vi "RT Video Server.vi"(11 "reader url":string) -> ()   [LabVIEW 2015]
uses:
  Controls/RT Streamer Queue element.ctl
  Controls/RT Streamer State.ctl
  RT Controls/Generic instruction typedef.ctl
  LP Globals.vi
  <vilib>/vision/NI_Vision_Development_Module.lvlib
  <resource>/objmgr/ni.dex.rc
  <vilib>/vision/Image Controls.llb/IMAQ Image.ctl
  IP Dev Area/IP results.ctl
panel:
  in  "Frames":u16
  in  "StartSave":bool
  out "error out":errorcluster
  out "output cluster":T1
  out "Frame Rate":dbl
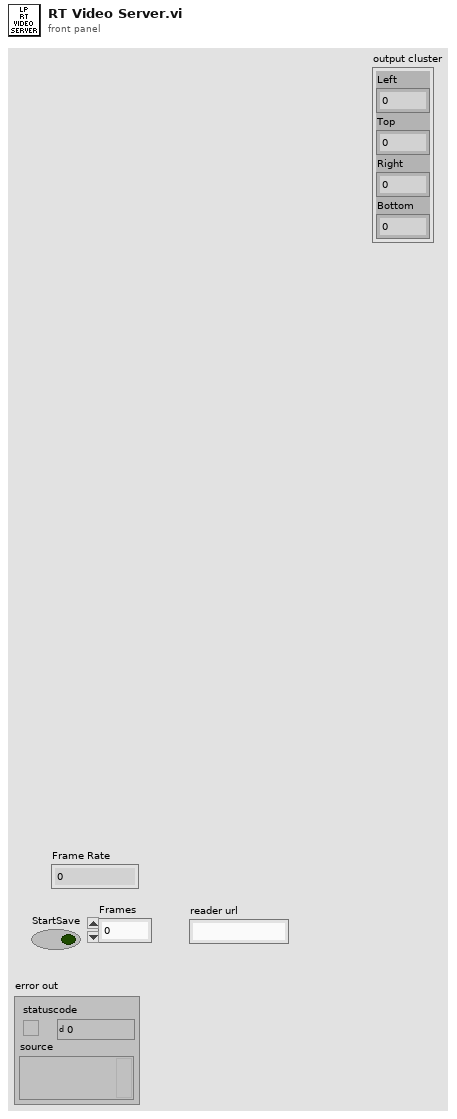
[diagram p1: front panel]
types:
  T1 = cluster{"Left":i32, "Top":i32, "Right":i32, "Bottom":i32}
  T2 = typedef "Image Type" = u32
  T3 = typedef "RT Streamer Queue element.ctl" = cluster{"CMD":T4, "Data":variant, "Error in":errorcluster}
  T4 = typedef "RT Streamer State.ctl" = enum16{"Init", "Idle", "Stream", "Listen", "SetRefrashRate", "SendCmdAck", "SendCmdDone", "SendSysState", "StartRecord", "Green Cordinates", "Error"}
  T5 = typedef "IMAQ Image.ctl" = refnum<image>
  T6 = typedef "Generic instruction typedef.ctl" = cluster{"CMD":string, "Data":variant}
  T7 = typedef "IP results.ctl" = cluster{"X":u16, "Y":u16, "A":dbl, "B":dbl, "Grade":u16, "Frame#":u16}
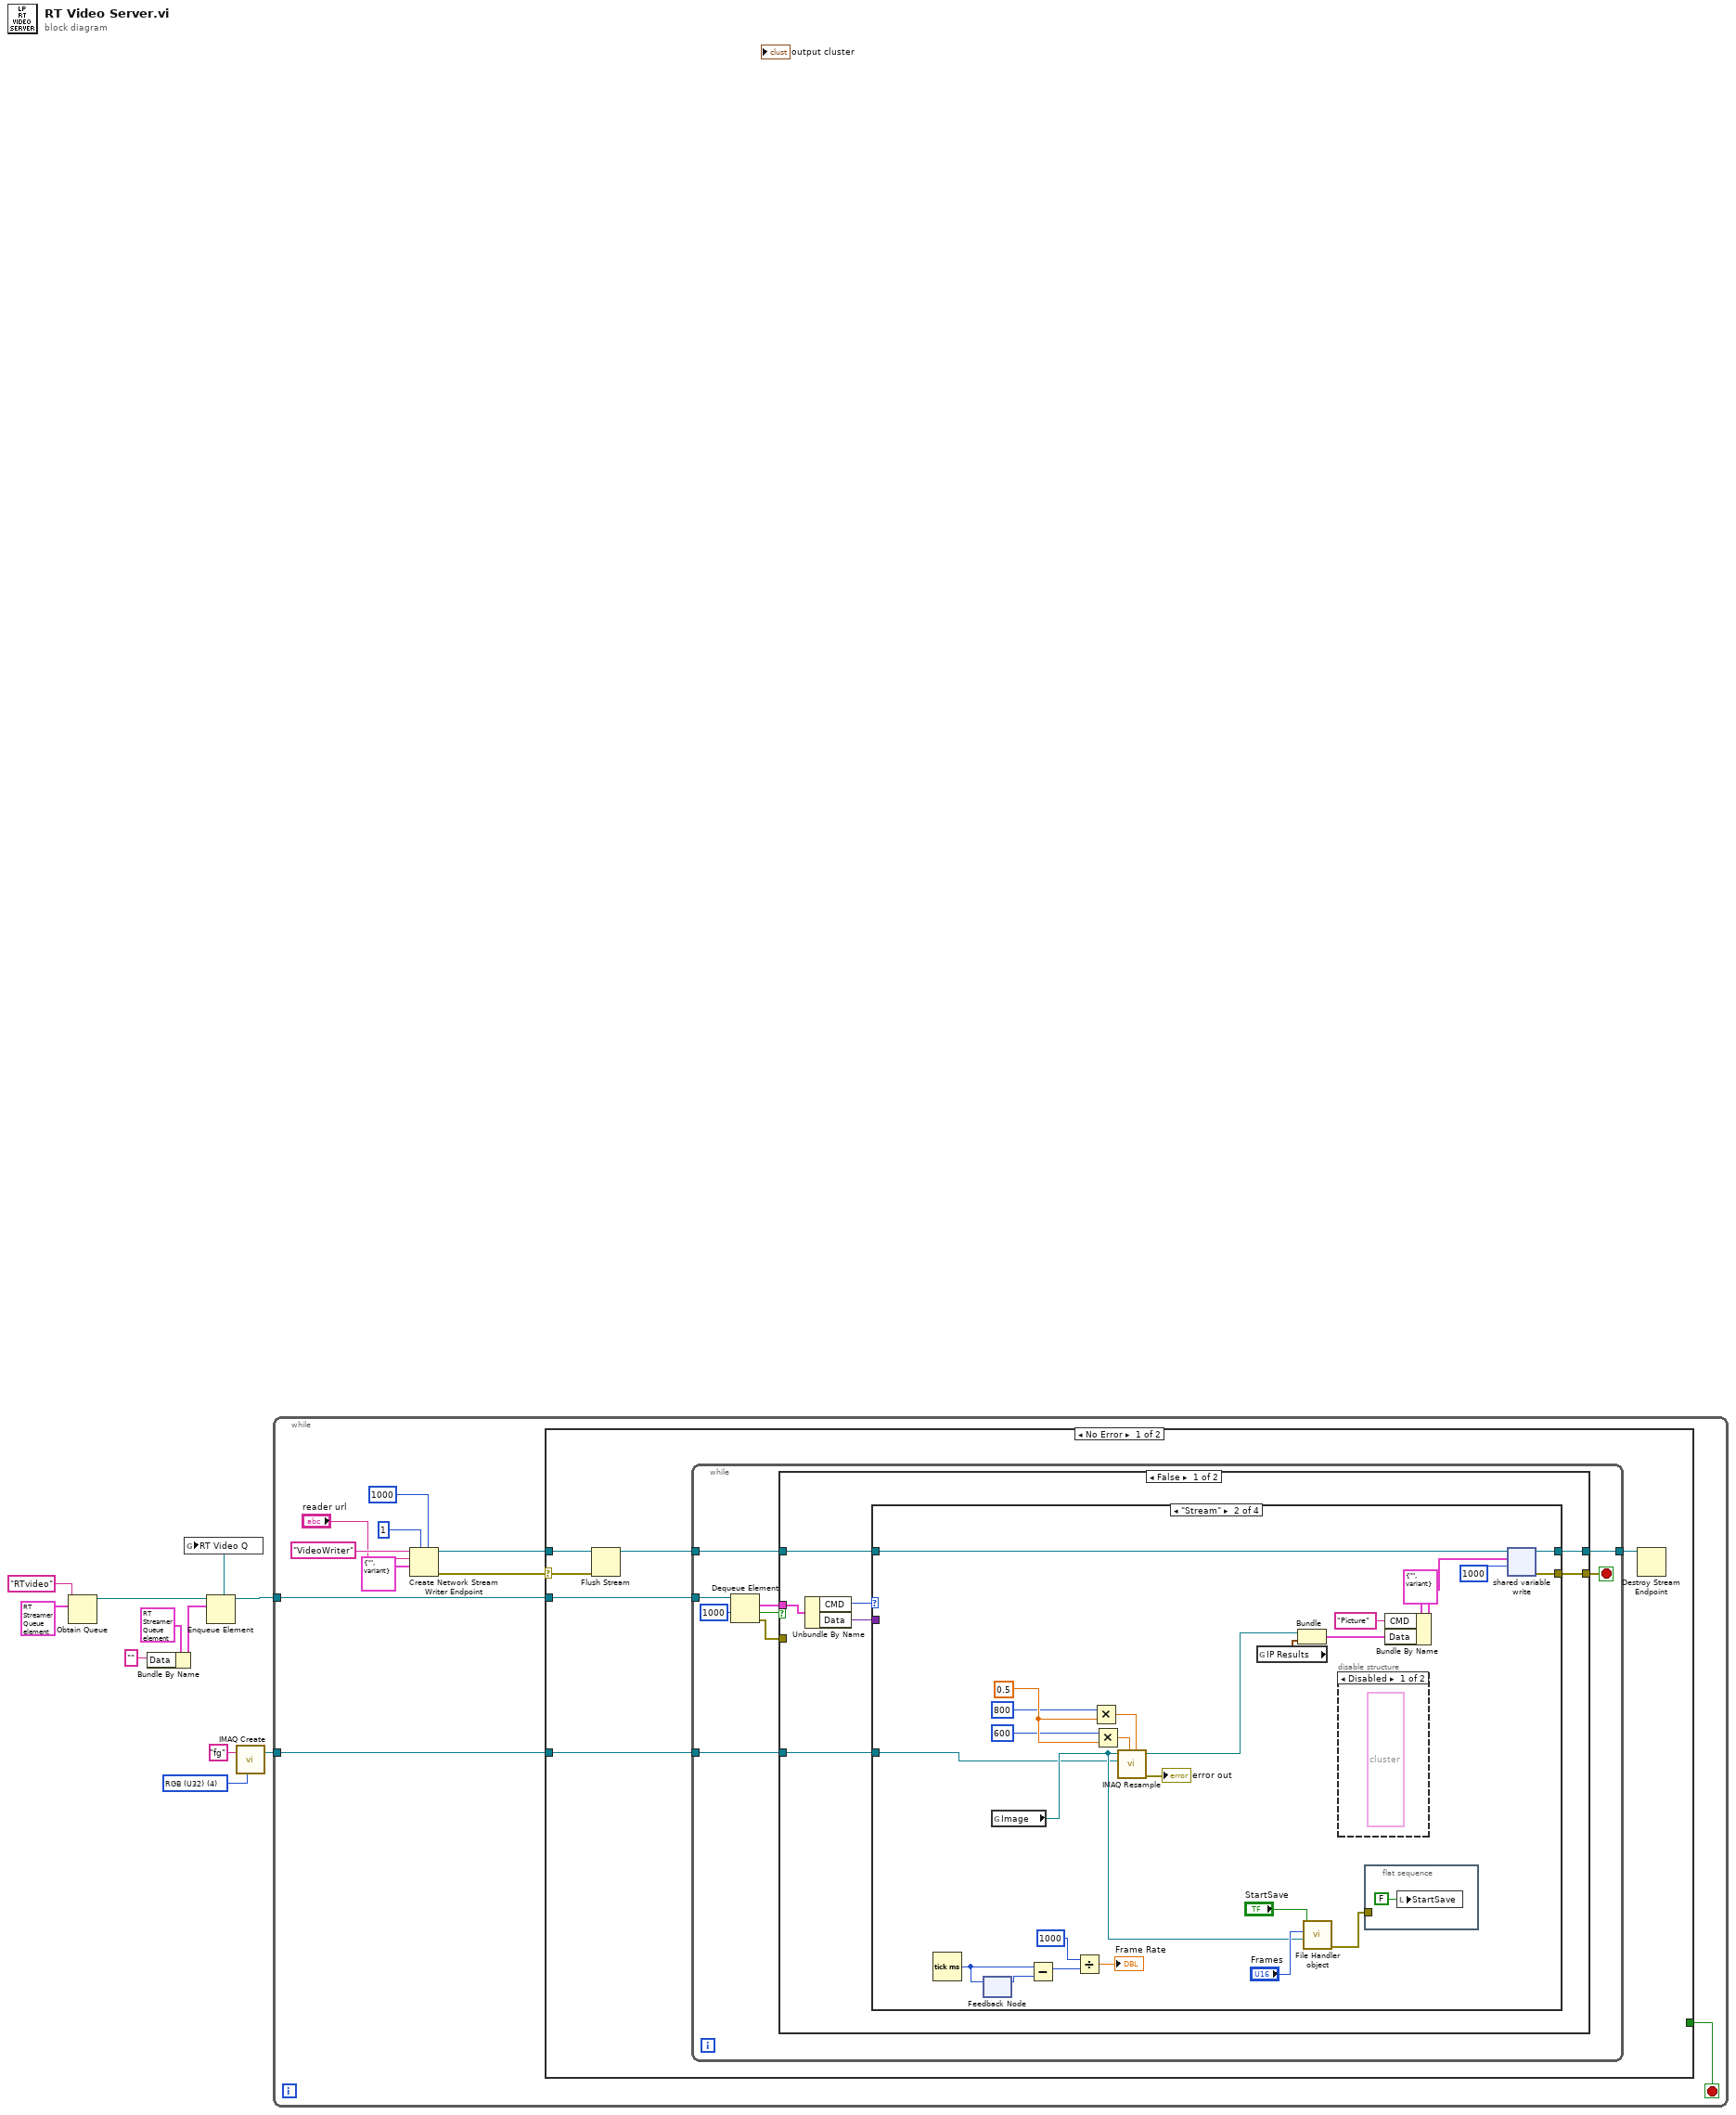
[diagram p0: block diagram]
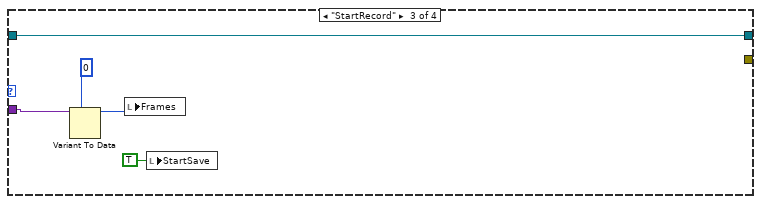
[diagram p4: hidden frame]
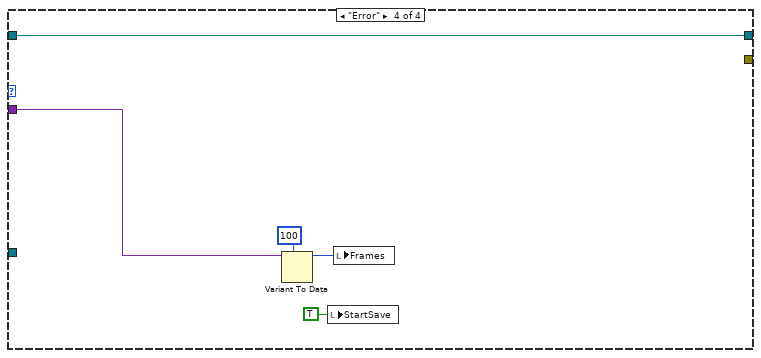
[diagram p5: hidden frame]
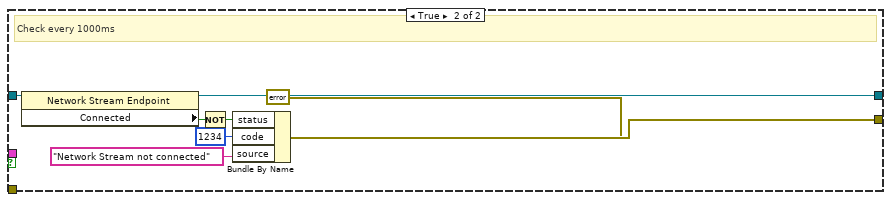
[diagram p6: hidden frame]
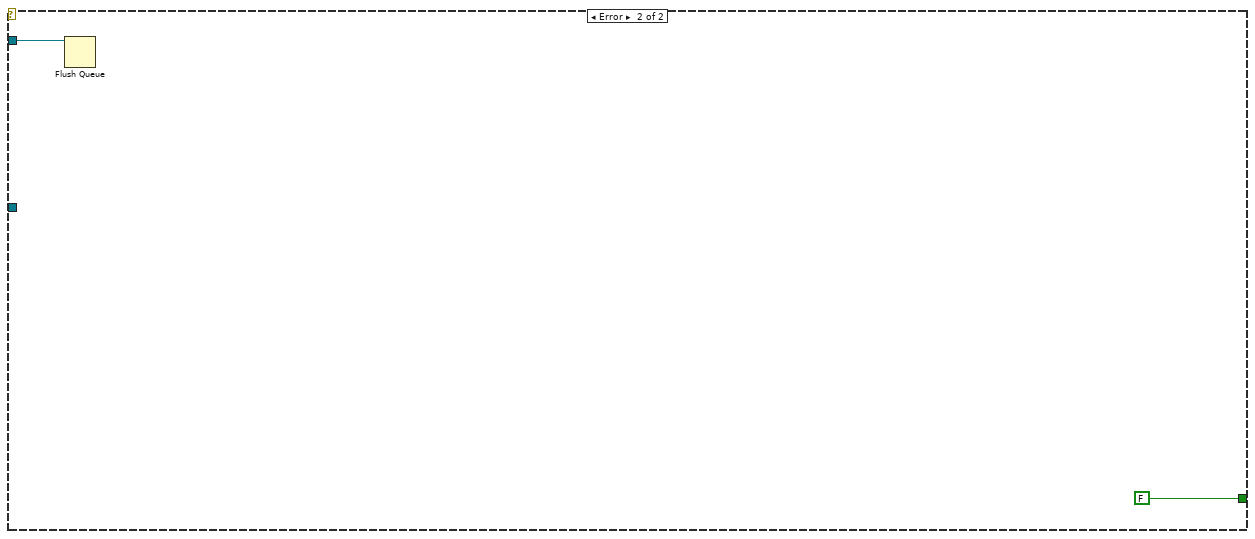
[diagram p7: hidden frame]
diagram:
  w3 = T2 4 items=["Grayscale (U8)", "Grayscale (I16)", "Grayscale (SGL)", "Complex (CSG)", "RGB (U32)", "HSL (U32)", "RGB (U64)", "Grayscale (U16)"] ("Image Type")
  n1 = Obtain Queue(name (unnamed)="RTvideo", element data type=T3 {"CMD"=enum."Init", "Data"=variant, "Error in"={"status"=FALSE, "code"=0, "source"=""}}) -> (queue out=w8:refnum<queue>)  [unwired: 3 in, 2 out]
  n2 = Bundle By Name(cluster=T3 {"CMD"=enum."Init", "Data"=variant, "Error in"={"status"=FALSE, "code"=0, "source"=""}} ("element"), "Data"="") -> (w6:T3)
  n3 = Enqueue Element(queue=w8, element=w6) -> (queue out=w2:refnum<queue>)  [unwired: 2 in, 2 out]
  n4 = global write "LP Globals.vi" "RT Video Q"(w2) -> ()
  n5 = call "IMAQ Create"("Image Name"="fg", "Image Type"=w3) -> ("New Image"=w1:T5)  [unwired: 3 in, 1 out]
  n6 = while {
    tunnel: w2 -> [w14]
    tunnel: w1 -> [w13]
    stop <- w20 stop-if-true
    n7 = Create Network Stream Writer Endpoint(5:1000 ("timeout in ms (-1)"), 7:1 ("writer buffer size"), 9:T6 {"CMD"="", "Data"=variant}, 10:"reader url", 11:"VideoWriter" ("reader url")) -> (0:w17:errorcluster, 3:w16:refnum<k21>)  [unwired: 2 in]
    n8 = case shown="No Error" w17 {
      selector: w17 -> [w21 _]
      tunnel: w16 -> [w26 _]
      tunnel: [_ FALSE ("Close")] -> w20
      tunnel: w14 -> [w25 w89]
      tunnel: w13 -> [w23 _]
      frame No Error {
        n9 = Flush Stream(8:w21, 11:w26) -> (3:w22:refnum<k21>)  [unwired: 2 in, 2 out]
        n10 = while {
          tunnel: w22 -> [w35]
          tunnel: w25 -> [w33]
          tunnel: [w29] -> w24
          tunnel: w23 -> [w28]
          stop <- w34 stop-if-true
          n11 = Dequeue Element(queue=w33, timeout in ms (-1)=1000) -> (element=w32:T3, timed out?=w30:bool, error out=w27:errorcluster)  [unwired: 1 in, 1 out]
          n12 = case shown="False" w30 {
            tunnel: w35 -> [w42 w88]
            tunnel: [w41 w87] -> w34
            tunnel: w32 -> [w40 _]
            tunnel: [w38 w81] -> w29
            tunnel: w28 -> [w36 _]
            tunnel: w27 -> [_ _]
            frame False {
              n13 = Unbundle By Name(w40) -> ("CMD"=w39:T4, "Data"=w37:variant)
              n14 = case shown="\"Stream\"" w39 {
                tunnel: w42 -> [w43 w69 w75 w76]
                tunnel: [_ w67 _ _] -> w41
                tunnel: [w43 w66 w75 w76] -> w38
                tunnel: w37 -> [_ _ w74 w77]
                tunnel: w36 -> [_ w52 _ _]
                frame Default {
                }
                frame "Stream" {
                  w51 = 0.5
                  n15 = Tick Count (ms)() -> (millisecond timer value=w55:u32)
                  n16 = feedback #1() -> (w56:u32)  [unwired: 1 in]
                  n17 = feedback-in #1(w55) -> ()
                  n18 = global read "LP Globals.vi" "Image"() -> (w62:T5)
                  n19 = Subtract(x=w55, y=w56) -> (x-y=w57:u32)
                  n20 = Divide(x=u32 1000, y=w57) -> (x/y=→"Frame Rate":dbl)
                  n21 = Multiply(x=800 ("Y Resolution"), y=w51) -> (x*y=w48:dbl)
                  n22 = Multiply(x=600 ("Y Resolution"), y=w51) -> (x*y=w47:dbl)
                  n23 = call "IMAQ Resample"("X Resolution"=w48, "Y Resolution"=w47, "Image Dst"=w52, "Image Src"=w62) -> ("error out"=→"error out":errorcluster, "Image Dst Out"=w46:T5)  [unwired: 6 in]
                  n24 = global read "LP Globals.vi" "IP Results"() -> (w45:T7)
                  n25 = Bundle("Image Dst Out"=w46, "IP Results"=w45) -> (w44:cluster{"Image Dst Out":T5, "IP Results":T7})  [unwired: 1 in]
                  n26 = call "File Handler object.vi"("Image"=w62, "Frames"="Frames", "Start"="StartSave") -> ("error out"=w65:errorcluster)  [unwired: 8 in]
                  n27 = disable-structure shown="Disabled" {
                    frame Disabled {
                      (unwired) cluster{"Image Dst Out":T5, "IP Results":T7} {"Image Dst Out"=refnum, "IP Results"={"X"=0, "Y"=0, "A"=0.0, "B"=0.0, "Grade"=0, "Frame#"=0}} ("output cluster")
                    }
                    frame Enabled {
                    }
                  }
                  n28 = flat-sequence {
                    tunnel: w65 -> [_]
                    frame #0 {
                      n29 = local write "StartSave"(FALSE ("StartSave")) -> ()
                    }
                  }
                  n30 = Bundle By Name(cluster=T6 {"CMD"="", "Data"=variant}, "CMD"="Picture", "Data"=w44) -> (w53:T6)
                  n31 = shared-variable-write(w69, w53, 1000 ("timeout ms (-1)")) -> (w66:refnum<k21>, w67:errorcluster)  [unwired: 1 in, 1 out]
                }
                frame "StartRecord" {
                  n32 = Variant To Data(type=u16 0 ("Frames"), Variant=w74) -> (data=w72:u16)  [unwired: 1 in, 1 out]
                  n33 = local write "Frames"(w72) -> ()
                  n34 = local write "StartSave"(TRUE ("StartSave")) -> ()
                }
                frame "Error" {
                  n35 = Variant To Data(type=u16 100 ("Frames"), Variant=w77) -> (data=w79:u16)  [unwired: 1 in, 1 out]
                  n36 = local write "StartSave"(TRUE ("StartSave")) -> ()
                  n37 = local write "Frames"(w79) -> ()
                }
              }
            }
            frame True {
              # "Check every 1000ms"
              n38 = property class="Network Stream Endpoint"(reference=w88) -> (reference out=w81:refnum<k21>, "Connected"=w86:bool)  [unwired: 1 in, 1 out]
              n39 = Not(x=w86) -> (.not. x?=w84:bool)
              n40 = Bundle By Name(cluster=errorcluster {"status"=FALSE, "code"=0, "source"=""} ("error IO"), "status"=w84, "code"=1234, "source"="Network Stream not connected") -> (w87:errorcluster)
            }
          }
        }
        n41 = Destroy Stream Endpoint(11:w24) -> ()  [unwired: 1 in, 1 out]
      }
      frame Error {
        n42 = Flush Queue(queue=w89) -> ()  [unwired: 1 in, 3 out]
      }
    }
  }
